vi "API Reference.vi"   [LabVIEW 2015]
uses:
  <vilib>/SLSC/SLSC.lvlib
  <vilib>/SLSC/Initialize Session with Devices.vi
  <resource>/objmgr/slsc.rc
  <vilib>/SLSC/Flatten Names (Device).vi
  <vilib>/SLSC/Set Device Property (Bool).vi
  <vilib>/SLSC/Get Device Property (Bool).vi
  <vilib>/SLSC/Unflatten Names (Device).vi
  <vilib>/SLSC/Set Phys Chan Property (Bool).vi
  <vilib>/SLSC/Get Phys Chan Property (Bool).vi
  <vilib>/SLSC/Commit Properties for Devices.vi
  <vilib>/SLSC/Execute Device Command.vi
  <vilib>/SLSC/Close Session.vi
  SLSC Interface.lvclass
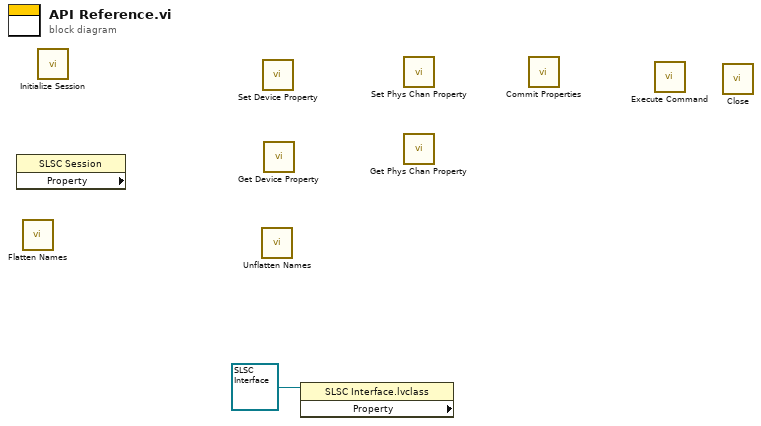
[diagram p0: block diagram]
diagram:
  n1 = property class="SLSC Session" props=[]() -> ()  [unwired: 2 in, 3 out]
  n2 = call-poly <vilib>:"Flatten Names.vi"() -> ()  [unwired: 14 in, 2 out]
  n3 = call-poly <vilib>:"Initialize Session.vi"() -> ()  [unwired: 14 in, 2 out]
  n4 = call-poly <vilib>:"Unflatten Names.vi"() -> ()  [unwired: 14 in, 2 out]
  n5 = call-poly <vilib>:"Set Device Property.vi"() -> ()  [unwired: 14 in, 2 out]
  n6 = call-poly <vilib>:"Get Device Property.vi"() -> ()  [unwired: 13 in, 3 out]
  n7 = property class="SLSC Interface.lvclass" props=[](reference=refnum<class "SLSC Interface.lvclass"> refnum ("SLSC Interface.lvclass")) -> ()  [unwired: 1 in, 3 out]
  n8 = call-poly <vilib>:"Set Phys Chan Property.vi"() -> ()  [unwired: 14 in, 2 out]
  n9 = call-poly <vilib>:"Get Phys Chan Property.vi"() -> ()  [unwired: 13 in, 3 out]
  n10 = call-poly <vilib>:"Commit Properties.vi"() -> ()  [unwired: 14 in, 2 out]
  n11 = call-poly <vilib>:"Execute Command.vi"() -> ()  [unwired: 14 in, 2 out]
  n12 = call-poly <vilib>:"Close.vi"() -> ()  [unwired: 15 in, 1 out]
